vi "WriteTextOnPicture.vi"(4 "颜色":u32(colorbox)=14418007, 6 "文本":string="123张哲zhang", 8 "user-specified font":T1={"Font Name:"="楷书", "Size"=16, "Strikeout?"=FALSE, "Italic?"=FALSE, "Underline?"=FALSE, "Outline?"=FALSE, "Shadow?"=FALSE, "Bold?"=FALSE} caption="字体", 9 "列索引":u32, 10 "行索引":u32, 11 "Origin Picture":picture) -> (3 "Picture Out":picture)   [LabVIEW 2012, in "WaveGraphX.xctl"]
uses:
  WaveGraphX.xctl
panel:
  # "输入 \n\n字体, \n字号, \n颜色, \n写入的行索引\n写入的列索引\n源图片"
  # "输出\n\n目的图片"
  # "画前要先清除对应行的原有的像素点, 否则会像素点重合"
  # "画前清除属性被关闭"
  # "大小 就是字体高度的点数\n但宽度就说不准了, 汉字较宽, 字母和数字较窄"
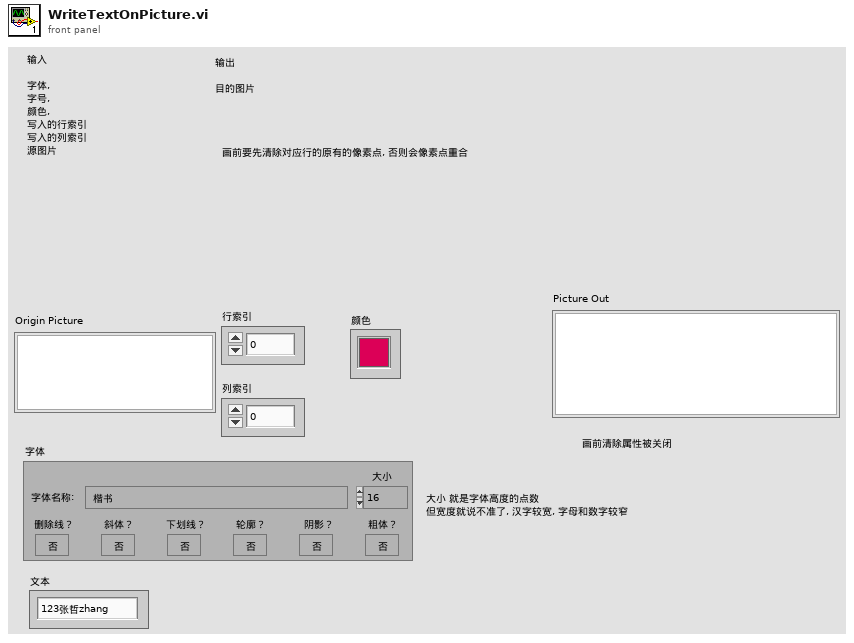
[diagram p1: front panel]
types:
  T1 = cluster{"Font Name:":string, "Size":i16, "Strikeout?":bool, "Italic?":bool, "Underline?":bool, "Outline?":bool, "Shadow?":bool, "Bold?":bool}
  T2 = enum16{"User-specified Font", "Application Font", "System Font", "Dialog Font"}
  T3 = cluster{"left_x":dbl, "left_y":dbl, "right_x":dbl, "right_y":dbl}
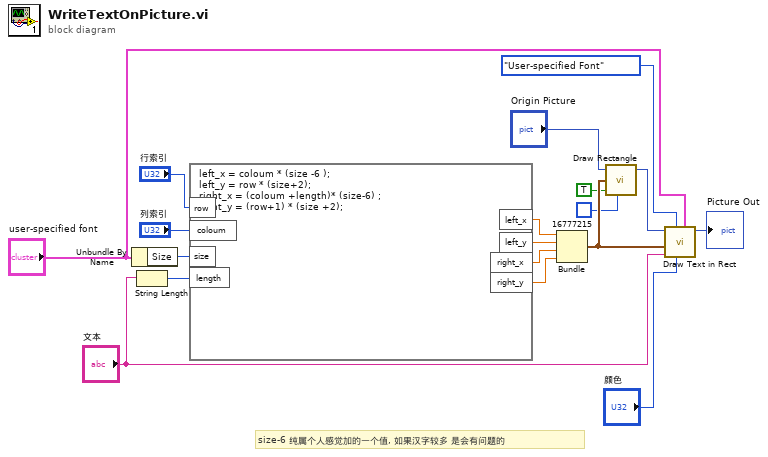
[diagram p0: block diagram]
diagram:
  # "size-6 纯属个人感觉加的一个值, 如果汉字较多 是会有问题的"
  n1 = Unbundle By Name("user-specified font") -> ("Size"=w11:i16)
  n2 = String Length(string="文本") -> (length=w10:i32)
  n3 = formula code="left_x = coloum * (size -6 ); \nleft_y = row * (size+2);\nright_x = (coloum +length)* (size-6) ;\nright_y = (row+1) * (size +2);"("row"="行索引", "coloum"="列索引", "size"=w11, "length"=w10) -> ("left_x"=w9:dbl, "left_y"=w8:dbl, "right_x"=w7:dbl, "right_y"=w6:dbl)
  n4 = Bundle("left_x"=w9, "left_y"=w8, "right_x"=w7, "right_y"=w6) -> (w4:T3)  [unwired: 1 in]
  n5 = call <vilib>:"Draw Rectangle.vi"("picture"="Origin Picture", "rect"=w4, "fill?(F)"=TRUE, "color(black)"=u32 16777215) -> ("new picture"=w1:picture)  [unwired: 5 in]
  n6 = call <vilib>:"Draw Text in Rect.vi"("[user-specified font]"="user-specified font", "text color(black)"="颜色", "desired font(Application)"=T2."User-specified Font", "text"="文本", "rect"=w4, "picture"=w1) -> ("new picture"=→"Picture Out":picture)  [unwired: 5 in]
